vi "Example.vi"() -> ()   [LabVIEW 2018, in "File Parsing Interface.lvlib" / "File Parsing Interface.lvclass"]
uses:
  File Parsing Interface.lvclass
  Plugins/String Database.lvlibp/String Database.lvclass
  Plugins/Measurement Data.lvlibp/Measurement Data.lvclass
panel:
  out "Values":string[][](array[string])
  out "error out":errorcluster
  in  "File to Parse":path=path "C:/Users/QFE3320 VM/Desktop/New Text Document.txt"
  in  "Directory of Plugins":path=path "C:/Sequence Automation/Classes/File Parsing/Interfaces"
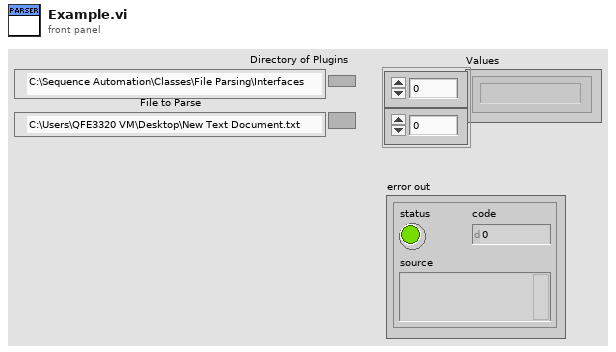
[diagram p1: front panel]
types:
  T1 = typedef "File Parsing Interface.lvlib/File Parsing Interface.lvclass/Parsed Measurement.ctl" = cluster{"Test Mode":string, "Measurement Data Out":refnum<class "Measurement Data.lvclass">}
  T2 = typedef "Measurement Data.lvlibp/Measurement Data.lvclass/Measurement Description.ctl" = cluster{"Measurement Sequence Position":T3, "Measurement Data":refnum<class "String Database.lvclass">, "Measurement Definition Entry":string}
  T3 = typedef "Measurement Data.lvlibp/Measurement Data.lvclass/Measurement Position.ctl" = enum16{"PreMeasurement", "MainMeasurement", "PostMeasurement"}
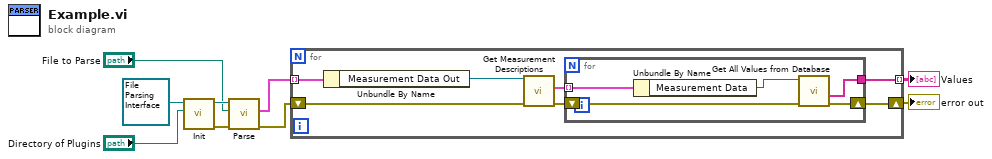
[diagram p0: block diagram]
diagram:
  n1 = call-dynamic "Init.vi"("Folder Path"="Directory of Plugins", "Plugin Framework In"=refnum<class "File Parsing Interface.lvclass"> refnum ("File Parsing Interface in")) -> ("Error Out"=w3:errorcluster, "Factory Plugin Framework out"=w2:refnum<class "File Parsing Interface.lvclass">)  [unwired: 8 in]
  n2 = call-dynamic "Parse.vi"("error in (no error)"=w3, "File to Parse"="File to Parse", "File Parsing Interface in"=w2) -> ("error out"=w6:errorcluster, "Measurements Out"=w9:T1[])  [unwired: 6 in, 1 out]
  n3 = for {
    tunnel: w9 -> [w14] mode=indexing
    shift-right: [w16] -> w5
    shift-left: w6 -> [w13]
    tunnel: [w15] -> w4 mode=indexing
    n4 = Unbundle By Name(w14) -> ("Measurement Data Out"=w10:refnum<class "Measurement Data.lvclass">)
    n5 = call "Get Measurement Descriptions.vi"("error in (no error)"=w13, "Measurement Data in"=w10) -> ("error out"=w12:errorcluster, "Measurement Step Descriptions"=w11:T2[])  [unwired: 7 in, 1 out]
    n6 = for {
      tunnel: [w20] -> w15
      shift-right: [w21] -> w16
      shift-left: w12 -> [w19]
      tunnel: w11 -> [w18] mode=indexing
      n7 = Unbundle By Name(w18) -> ("Measurement Data"=w17:refnum<class "String Database.lvclass">)
      n8 = call "Get All Values from Database.vi"("error in (no error)"=w19, "String Database in"=w17) -> ("error out"=w21:errorcluster, "Values"=w20:string[])  [unwired: 6 in, 2 out]
    }
  }
  "error out" <- w5
  "Values" <- w4
